vi "ESM-xx50.vi"(4 "parity":u16(ring) items=["None", "Odd", "Even"], 6 "Slave ID":u8=1, 8 "error in (no error)":errorcluster, 10 "baud rate (9600)":u32=9600, 11 "Serial Port":string) -> (0 "error out":errorcluster, 3 "EMKO Out":refnum<class "ESM-xx50.lvclass">)   [LabVIEW 2022 SP3, in "EMKO.lvlib" / "ESM-xx50.lvclass"]
uses:
  ESM-xx50.lvclass
  ESM-xx50.lvclass/ESM-xx50.ctl
  <vilib>/Modbus/master/Create Master Instance (Serial).vi
  <vilib>/Modbus/master/Modbus Master.lvclass
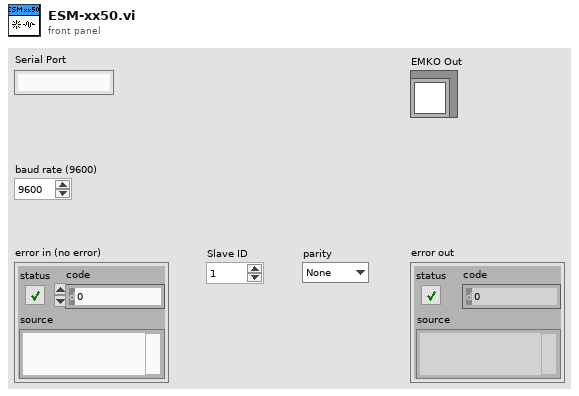
[diagram p1: front panel]
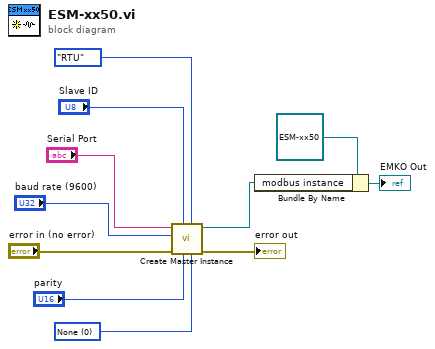
[diagram p0: block diagram]
diagram:
  w6 = u16 0 items=["None", "XON/XOFF", "RTS/CTS", "XON/XOFF & RTS/CTS", "DTR/DSR", "XON/XOFF & DTR/DSR"] ("flow control (None)")
  n1 = call-poly <vilib>:"Create Master Instance.vi"("flow control (None)"=w6, "serial type"=enum16{"RTU", "ASCII"}."RTU", "parity (Even)"="parity", "unit ID"="Slave ID", "error in (no error)"="error in (no error)", "baud rate (9600)"="baud rate (9600)", "VISA resource name"="Serial Port") -> ("error out"=→"error out":errorcluster, "serial master instance"=w1:refnum<class "Modbus Master.lvclass">)  [unwired: 3 in]
  n2 = Bundle By Name(cluster=refnum<class "ESM-xx50.lvclass"> refnum ("EMKO Out"), "modbus instance"=w1) -> (→"EMKO Out":refnum<class "ESM-xx50.lvclass">)
